vi "SVFA Zoom FFT Spectrum (Real-Im).vi"   [LabVIEW 2017]
doc: "Computes the zoom FFT spectrum of <B>scaled signal [EU]</B> and <B>zoom settings</B>. Zoom FFT results are returned as real part and imaginary part. Data accumulates each time this VI is called. However, it returns a new spectrum only when sufficient data accumulates. Indicators and subsequent processing should only be called when <B>new spectrum available</B> is TRUE. Wire data to the <B>scaled signal [EU]</B> input to determine the polymorphic instance to use or manually select the instance."
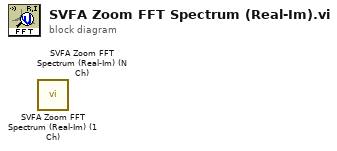
[diagram p0: block diagram]
diagram:
  n1 = call <vilib>:"SVFA Zoom FFT Spectrum (Real-Im) (1 Ch).vi"() -> ()  [unwired: 12 in, 8 out]
  n2 = call <vilib>:"SVFA Zoom FFT Spectrum (Real-Im) (N Ch).vi"() -> ()  [unwired: 12 in, 8 out]
